vi "AlliGator Update Displayed Image.vi"(7 "Bkgd Image Subtraction?":bool, 8 "Error In":errorcluster, 9 "Sum Image Ref":T1, 11 "Displayed Image Ref":T1) -> (0 "Error Out":errorcluster, 3 "Displayed Image Ref":T1)   [LabVIEW 2021, in "AlliGator Source Image.lvlib"]
doc: "Updates displayed image if background correction is not expected to follow immediately after."
uses:
  AlliGator Source Image.lvlib
  <vilib>/vision/Image Controls.llb/IMAQ Image.ctl
panel:
  # "see the AlliGator License on the block diagram (Ctrl+E or Window:Show Block Diagram)"
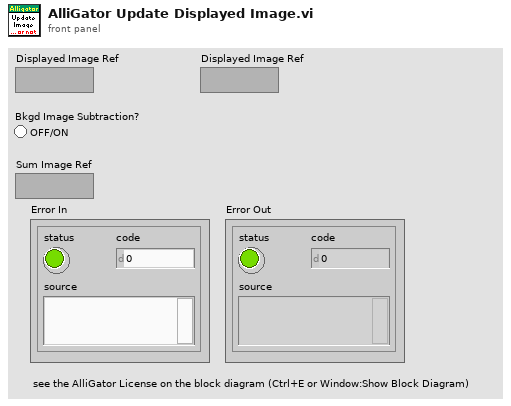
[diagram p1: front panel]
types:
  T1 = typedef "IMAQ Image.ctl" = refnum<image>
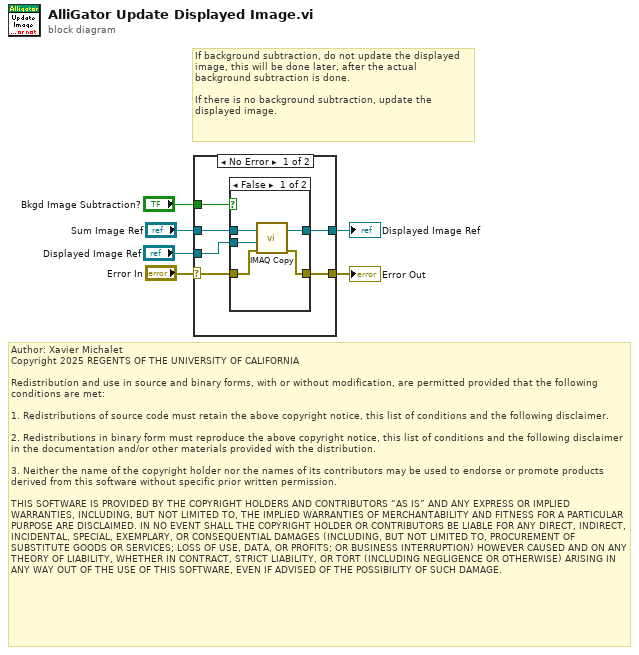
[diagram p0: block diagram]
diagram:
  # "Author: Xavier Michalet\nCopyright 2025 REGENTS OF THE UNIVERSITY OF CALIFORNIA\n\nRedistribution and use in source and binary forms, with or without modification, are permitted provided that the following conditions are met:\n\n1. Redistributions of source code must retain the above copyright notice, this list of conditions and the following disclaimer.\n\n2. Redistributions in binary form must reproduce the above copyright notice, this list of conditions and the following disclaimer in the documentation and/or other materials provided with the distribution.\n\n3. Neither the name of the copyright holder nor the names of its contributors may be used to endorse or promote products derived from this software without specific prior written permission.\n\nTHIS SOFTWARE IS PROVIDED BY THE COPYRIGHT HOLDERS AND CONTRIBUTORS “AS IS” AND ANY EXPRESS OR IMPLIED WARRANTIES, INCLUDING, BUT NOT LIMITED TO, THE IMPLIED WARRANTIES OF MERCHANTABILITY AND FITNESS FOR A PARTICULAR PURPOSE ARE DISCLAIMED. IN NO EVENT SHALL THE COPYRIGHT HOLDER OR CONTRIBUTORS BE LIABLE FOR ANY DIRECT, INDIRECT, INCIDENTAL, SPECIAL, EXEMPLARY, OR CONSEQUENTIAL DAMAGES (INCLUDING, BUT NOT LIMITED TO, PROCUREMENT OF SUBSTITUTE GOODS OR SERVICES; LOSS OF USE, DATA, OR PROFITS; OR BUSINESS INTERRUPTION) HOWEVER CAUSED AND ON ANY THEORY OF LIABILITY, WHETHER IN CONTRACT, STRICT LIABILITY, OR TORT (INCLUDING NEGLIGENCE OR OTHERWISE) ARISING IN ANY WAY OUT OF THE USE OF THIS SOFTWARE, EVEN IF ADVISED OF THE POSSIBILITY OF SUCH DAMAGE."
  # "If background subtraction, do not update the displayed image, this will be done later, after the actual background subtraction is done.\n\nIf there is no background subtraction, update the displayed image."
  n1 = case shown="No Error" "Error In" {
    selector: "Error In" -> [w8 w20]
    tunnel: "Displayed Image Ref" -> [w12 w21]
    tunnel: [w11 w21] -> w5
    tunnel: "Sum Image Ref" -> [w10 _]
    tunnel: [w9 w20] -> w3
    tunnel: "Bkgd Image Subtraction?" -> [w7 _]
    frame No Error {
      n2 = case shown="False" w7 {
        tunnel: [w17 w19] -> w11
        tunnel: w8 -> [w16 w18]
        tunnel: w12 -> [w15 w19]
        tunnel: w10 -> [w14 _]
        tunnel: [w13 w18] -> w9
        frame False {
          n3 = call "IMAQ Copy"("error in (no error)"=w16, "Image Dst"=w15, "Image Src"=w14) -> ("error out"=w13:errorcluster, "Image Dst Out"=w17:T1)  [unwired: 3 in]
        }
        frame True {
        }
      }
    }
    frame Error {
    }
  }
  "Displayed Image Ref" <- w5
  "Error Out" <- w3
